vi "Initialize hitcharts.vi"(7 "Hit charts bottom":T1, 9 "Hit charts top":T1, 11 "error in":errorcluster, 12 "Resolution(s)":dbl) -> (4 "hit charts refnum cluster":T2, 15 "error out":errorcluster)   [LabVIEW 2016]
uses:
  Typedefs/Hit chart cluster refnum.ctl
  Global Variables/Scintillator IDs.vi
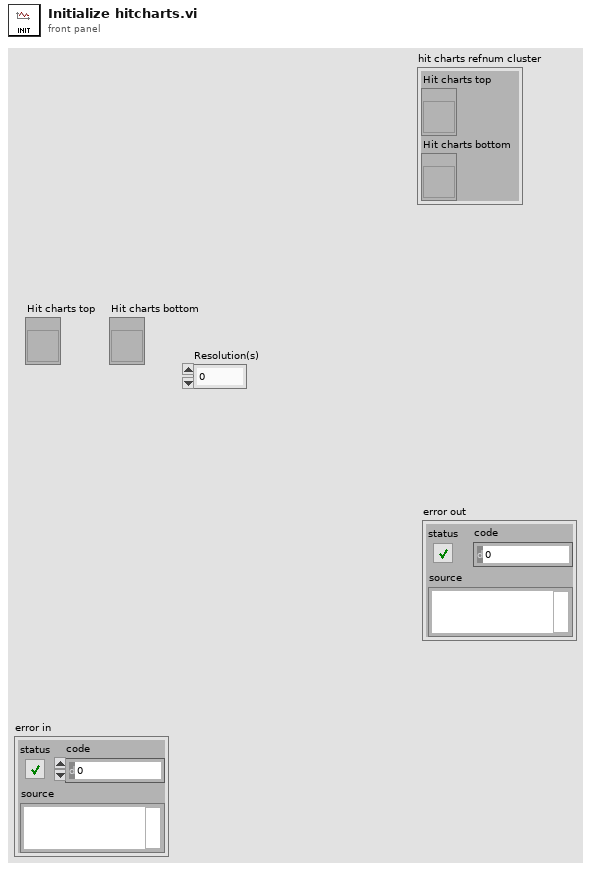
[diagram p1: front panel]
types:
  T1 = typedef "Hit chart cluster refnum.ctl" = refnum<vi>
  T2 = cluster{"Hit charts top":T1, "Hit charts bottom":T1}
  T3 = cluster{"Total hits":dbl, "Ratio":dbl, "Non-coincidences":dbl, "Coincidences":dbl}
  T4 = cluster{"Total hits":dbl, "Ratio":dbl, "Non-coincidences":dbl, "Coincidences":dbl}[]
  T5 = typedef "HitChart refnum.ctl" = refnum<vi>
  T6 = typedef "HitChart.ctl" = cluster{"Waveform Chart":cluster{"Coincidences":dbl, "Non-coincidences":dbl, "Ratio":dbl, "Total hits":dbl}[], "Last update timestamp":timestamp, "Resolution(s)":dbl, "nondisplayed coincs":i32, "nondisplayed noncoincs":i32, "Last upd":i64, "ID":i8}
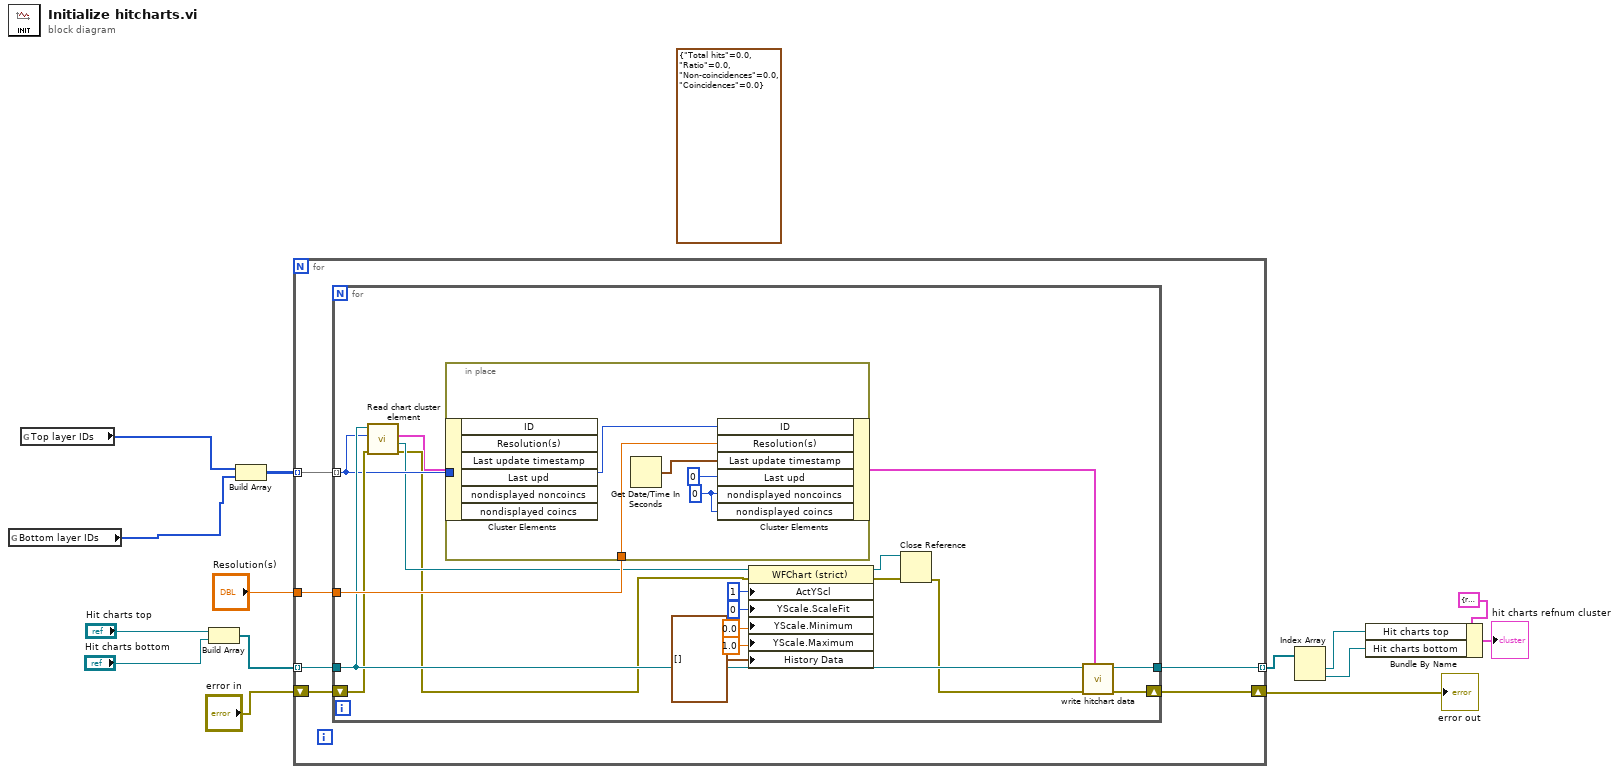
[diagram p0: block diagram]
diagram:
  (unwired) T3 {"Total hits"=0.0, "Ratio"=0.0, "Non-coincidences"=0.0, "Coincidences"=0.0}
  n1 = global read "Scintillator IDs.vi" "Bottom layer IDs"() -> (w7:i8[])
  n2 = global read "Scintillator IDs.vi" "Top layer IDs"() -> (w8:i8[])
  n3 = Build Array("Hit charts top", "Hit charts bottom") -> (w11:T1[])
  n4 = Build Array(w8, w7) -> (w9:i8[][])
  n5 = for {
    tunnel: w9 -> [w16] mode=indexing
    shift-right: [w19] -> w6
    shift-left: "error in" -> [w20]
    tunnel: w11 -> [w18] mode=indexing
    tunnel: [w17] -> w4 mode=indexing
    tunnel: "Resolution(s)" -> [w15]
    n6 = for {
      tunnel: w16 -> [w32] mode=indexing
      shift-right: [w38] -> w19
      shift-left: w20 -> [w33]
      tunnel: w18 -> [w34]
      tunnel: [w37] -> w17
      tunnel: w15 -> [w35]
      n7 = call "Read chart cluster element.vi"("error in (no error)"=w33, "Channel"=w32, "Chart cluster"=w34) -> ("error out"=w26:errorcluster, "Chart ref"=w27:T5, "Chart cluster"=w21:T6)  [unwired: 5 in, 1 out]
      n8 = in-place {
        in-place-border: w32 -> [w43]
        in-place-border: w35 -> [w42]
        w39 = 0 ("nondisplayed noncoincs")
        n9 = in-place-cluster #1(w21) -> ()  [unwired: 6 out]
        n10 = Get Date/Time In Seconds() -> (seconds since 1Jan1904=w41:timestamp)
        n11 = in-place-cluster #1("ID"=w43, "Resolution(s)"=w42, "Last update timestamp"=w41, "Last upd"=i64 0, "nondisplayed noncoincs"=w39, "nondisplayed coincs"=w39) -> (w36:T6)
      }
      n12 = property class="WFChart (strict)"(reference=w27, error in=w26, "ActYScl"=1 ("Active Y Scale"), "YScale.ScaleFit"=u8 0 ("Y Scale.Scale Fit"), "YScale.Minimum"=0.0 ("Y Scale.Range:Minimum"), "YScale.Maximum"=1.0 ("Y Scale.Range:Maximum"), "History Data"=T4 []) -> (reference out=w25:T5, error out=w24:errorcluster)
      n13 = Close Reference(reference=w25, error in (no error)=w24) -> (error out=w23:errorcluster)
      n14 = call "write hitchart data.vi"("Histogram cluster"=w36, "error in (no error)"=w23, "Hit charts"=w34) -> ("error out"=w38:errorcluster, "Hit charts"=w37:T1)  [unwired: 7 in]
    }
  }
  "error out" <- w6
  n15 = Index Array(array=w4) -> (element #1=w3:T1, element #2=w2:T1)  [unwired: 2 in]
  n16 = Bundle By Name(cluster=T2 {"Hit charts top"=refnum, "Hit charts bottom"=refnum}, "Hit charts top"=w3, "Hit charts bottom"=w2) -> (→"hit charts refnum cluster":T2)
